vi "DigitalInput-Driver.vi"(3 "error in (no error)":errorcluster, 4 "Configuration":T1={"Lines"=["6289/port1/line0", "6289/port1/line1", "6289/port1/line2", "6289/port1/line3", "6289/port1/line4", "6289/port1/line5", "6289/port1/line6", "6289/port1/line7"], "Refresh period (ms)"=0}, 5 "Command":enum16{"Refresh", "Start", "Stop"}(ring)) -> (0 "error out":errorcluster, 2 "DigitalInput":T2)   [LabVIEW 2015]
doc: "Input driver for digital input lines. See also: DigitalInput-Daemon.vi\n\nThis VI has 3 different functions:\n\n\"Refresh\" returns the current state of the digital inputs in the output cluster \"DigitalInput\", which contains 3 boolean arrays: \"State\" (the current state of the line), \"Rising\" (whether a rising edge occurred since last refresh), and \"Falling\" (whether a falling edge occurred since last refresh). The \"Configuration\" input is unused.\n\n\"Start\" starts the daemon running. \"Configuration\" is a cluster containing \"Lines\" (the I/O lines to check; this will be one-to-one with the boolean arrays returned by the \"Refresh\" command) and \"Update period\" (the # of ms between Poller update cycles). The \"DigitalInput\" output cluster is undefined and should not be used.\n\n\"Stop\" stops the daemon and releases the references. The \"Configuration\" input are unused. The \"DigitalInput\" output cluster is undefined and should not be used."
uses:
  DigitalInput-DataCluster.ctl
  DigitalInput-Configuration.ctl
panel:
  out "Data":T3
  out "stop":bool
  # "Internal data that will be accessed by the daemon"
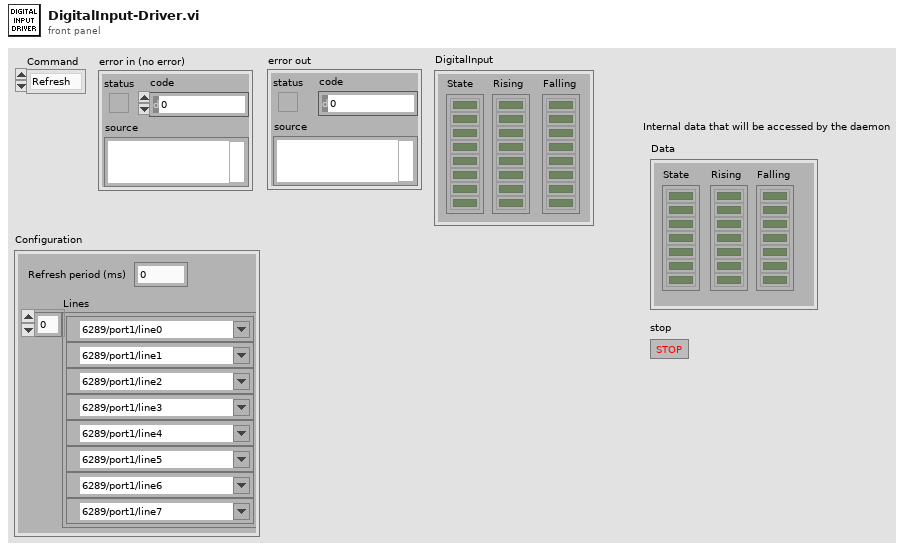
[diagram p1: front panel]
types:
  T1 = typedef "DigitalInput-Configuration.ctl" = cluster{"Lines":tag[], "Refresh period (ms)":u32}
  T2 = typedef "DigitalInput-DataCluster.ctl" = cluster{"Falling":bool[], "Rising":bool[], "State":bool[]}
  T3 = cluster{"State":bool[], "Rising":bool[], "Falling":bool[]}
  T4 = typedef "Semaphore RefNum" = refnum<k1>
  T5 = cluster{"Stop Refnum":refnum<vi>, "Data Refnum":refnum<vi>, "semaphore":T4}
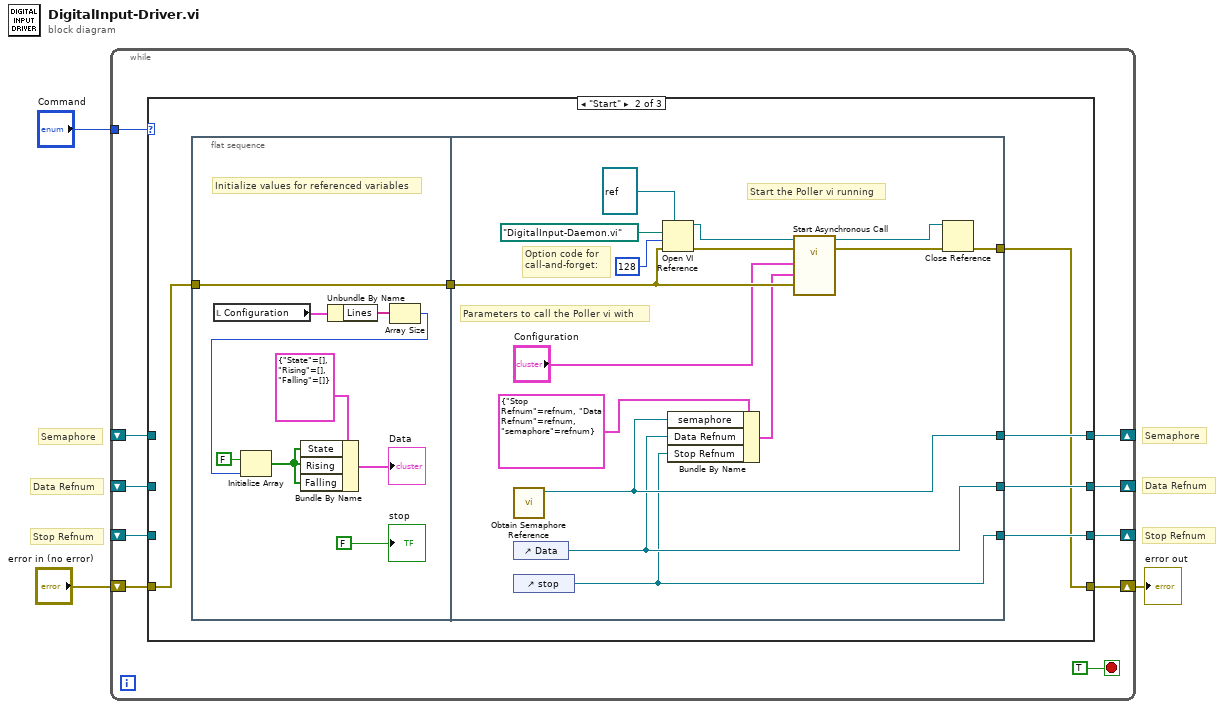
[diagram p0: block diagram]
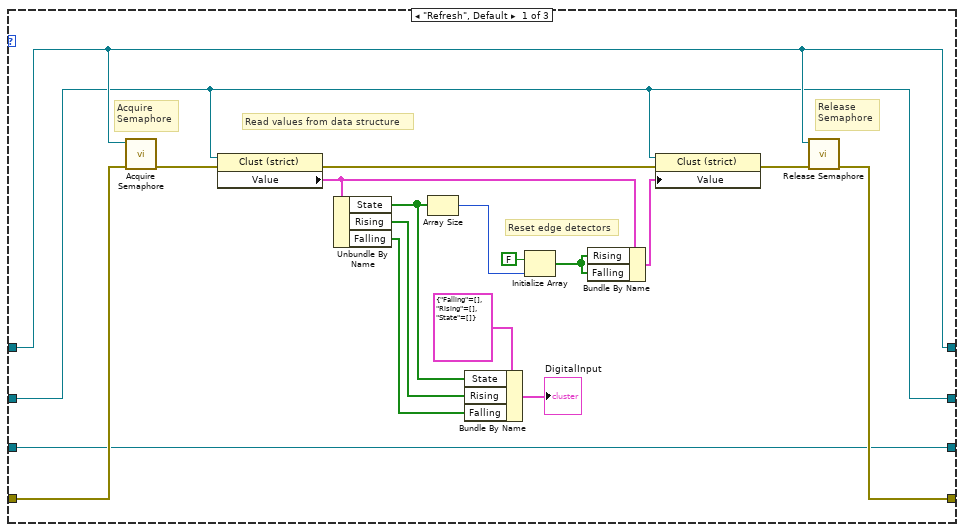
[diagram p2: hidden frame]
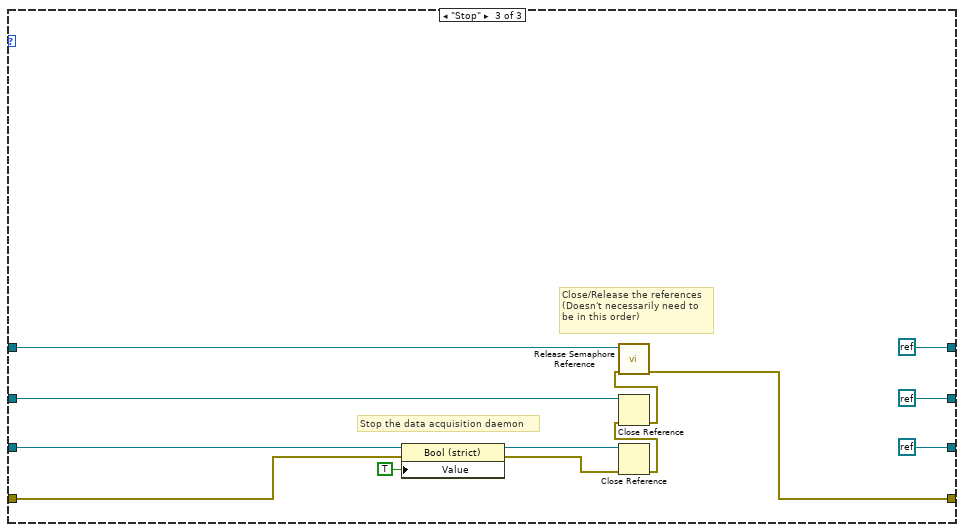
[diagram p3: hidden frame]
diagram:
  # "Stop Refnum"
  # "Data Refnum"
  # "Semaphore"
  # "Stop Refnum"
  # "Data Refnum"
  # "Semaphore"
  n1 = while {
    tunnel: "Command" -> [w12]
    shift-right: [w11] -> _
    shift-left: _ -> [w8]
    shift-right: [w10] -> _
    shift-left: _ -> [w7]
    shift-right: [w9] -> _
    shift-left: _ -> [w6]
    shift-right: [w4] -> w1
    shift-left: "error in (no error)" -> [w5]
    stop <- TRUE stop-if-true
    n2 = case shown="\"Start\"" w12 {
      tunnel: [w26 w37 refnum<k0> refnum] -> w11
      tunnel: [w25 w36 refnum<k0> refnum] -> w10
      tunnel: [w19 w35 refnum<k0> refnum] -> w9
      tunnel: w8 -> [w26 _ w72]
      tunnel: w7 -> [w25 _ w71]
      tunnel: w6 -> [w19 _ w70]
      tunnel: w5 -> [w20 w32 w69]
      tunnel: [w21 w34 w65] -> w4
      frame "Refresh", Default {
        # "Release\nSemaphore"
        # "Reset edge detectors"
        # "Read values from data structure"
        # "Acquire\nSemaphore"
        n3 = call <vilib>:"Acquire Semaphore.vi"("error in (no error)"=w20, "semaphore"=w26) -> ("error out"=w24:errorcluster)  [unwired: 3 in, 2 out]
        n4 = property class="Clust (strict)"(reference=w25, error in=w24) -> (error out=w23:errorcluster, "Value"=w31:T3)  [unwired: 1 out]
        n5 = Unbundle By Name(w31) -> ("State"=w18:bool[], "Rising"=w17:bool[], "Falling"=w16:bool[])
        n6 = Array Size(array=w18) -> (size(s)=w30:i32)
        n7 = Bundle By Name(cluster=T2 {"Falling"=[], "Rising"=[], "State"=[]} ("DigitalInput"), "State"=w18, "Rising"=w17, "Falling"=w16) -> (→"DigitalInput":T2)
        n8 = Initialize Array(FALSE, w30) -> (w28:bool[])
        n9 = Bundle By Name(cluster=w31, "Rising"=w28, "Falling"=w28) -> (w29:T3)
        n10 = property class="Clust (strict)"(reference=w25, error in=w23, "Value"=w29) -> (error out=w22:errorcluster)  [unwired: 1 out]
        n11 = call <vilib>:"Release Semaphore.vi"("error in (no error)"=w22, "semaphore"=w26) -> ("error out"=w21:errorcluster)  [unwired: 4 in, 1 out]
      }
      frame "Start" {
        n12 = flat-sequence {
          tunnel: [w41] -> w33
          tunnel: w32 -> [w41]
          tunnel: [w51] -> w37
          tunnel: [w50] -> w36
          tunnel: [w49] -> w35
          tunnel: [w54] -> w34
          tunnel: w33 -> [w53]
          frame #0 {
            # "Initialize values for referenced variables"
            n13 = local read "Configuration"() -> (w38:T1)
            n14 = Unbundle By Name(w38) -> ("Lines"=w40:tag[])
            n15 = Array Size(array=w40) -> (size(s)=w39:i32)
            n16 = Initialize Array(FALSE ("Boolean"), w39) -> (w44:bool[])
            n17 = Bundle By Name(cluster=T3 {"State"=[], "Rising"=[], "Falling"=[]} ("Data"), "State"=w44, "Rising"=w44, "Falling"=w44) -> (→"Data":T3)
            "stop" <- FALSE ("stop")
          }
          frame #1 {
            # "Start the Poller vi running"
            # "Option code for\ncall-and-forget:"
            # "Parameters to call the Poller vi with"
            n18 = call <vilib>:"Obtain Semaphore Reference.vi"() -> ("semaphore"=w51:T4)  [unwired: 5 in, 2 out]
            n19 = control-ref of="Data"() -> (w50:refnum<vi>)
            n20 = control-ref of="stop"() -> (w49:refnum<vi>)
            n21 = Open VI Reference(type specifier VI Refnum (for type only)=refnum<vi> refnum, vi path=path "DigitalInput-Daemon.vi", options=128, error in (no error)=w53) -> (vi reference=w59:refnum<vi>, error out=w58:errorcluster)  [unwired: 2 in]
            n22 = Bundle By Name(cluster=T5 {"Stop Refnum"=refnum, "Data Refnum"=refnum, "semaphore"=refnum} ("References"), "semaphore"=w51, "Data Refnum"=w50, "Stop Refnum"=w49) -> (w48:T5)
            n23 = call-by-ref "Start Asynchronous Call"(reference=w59, error in=w58, "error in"=w53, "References"=w48, "Configuration"="Configuration") -> (reference out=w55:refnum<vi>, error out=w56:errorcluster)  [unwired: 2 in, 1 out]
            n24 = Close Reference(reference=w55, error in (no error)=w56) -> (error out=w54:errorcluster)
          }
        }
      }
      frame "Stop" {
        # "Close/Release the references\n(Doesn't necessarily need to \nbe in this order)"
        # "Stop the data acquisition daemon"
        n25 = property class="Bool (strict)"(reference=w70, error in=w69, "Value"=TRUE) -> (reference out=w74:refnum<vi>, error out=w68:errorcluster)
        n26 = Close Reference(reference=w74, error in (no error)=w68) -> (error out=w67:errorcluster)
        n27 = Close Reference(reference=w71, error in (no error)=w67) -> (error out=w66:errorcluster)
        n28 = call <vilib>:"Release Semaphore Reference.vi"("error in (no error)"=w66, "semaphore"=w72) -> ("error out"=w65:errorcluster)  [unwired: 8 in, 1 out]
      }
    }
  }
  "error out" <- w1
